vi "Write Buffer Size.vi"(10 "Buffer Size":i32=4096, 11 "Network Stream in":refnum<class "Network Stream.lvclass">) -> (3 "Network Stream out":refnum<class "Network Stream.lvclass">)   [LabVIEW 2020, in "Network Stream.lvclass"]
doc: "Use this VI to specify the buffer size for this endpoint of the network stream."
uses:
  Network Stream.lvclass
  Network Stream.lvclass/Network Stream.ctl
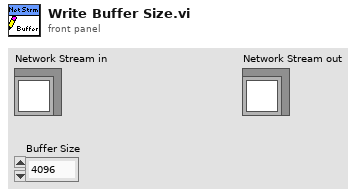
[diagram p1: front panel]
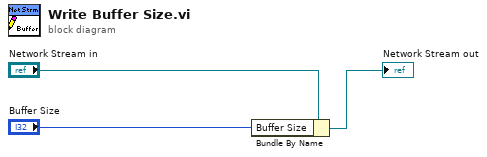
[diagram p0: block diagram]
diagram:
  n1 = Bundle By Name(cluster="Network Stream in", "Buffer Size"="Buffer Size") -> (→"Network Stream out":refnum<class "Network Stream.lvclass">)
